vi "Process_day_file_strat.vi"(2 "Filename":path=path "/G3_3 HD/EnFlo Data/Oct_2000/3_Oct") -> (6 "Day KW Hrs":dbl, 7 "Night KWHrs":dbl format="%.2f", 10 "Time":dbl)   [LabVIEW 2010]
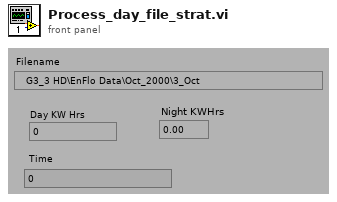
[diagram p1: front panel]
types:
  T1 = cluster{"second":i32, "minute":i32, "hour":i32, "day of month":i32, "month":i32, "year":i32, "day of week":i32, "day of year":i32, "is DST":i32}
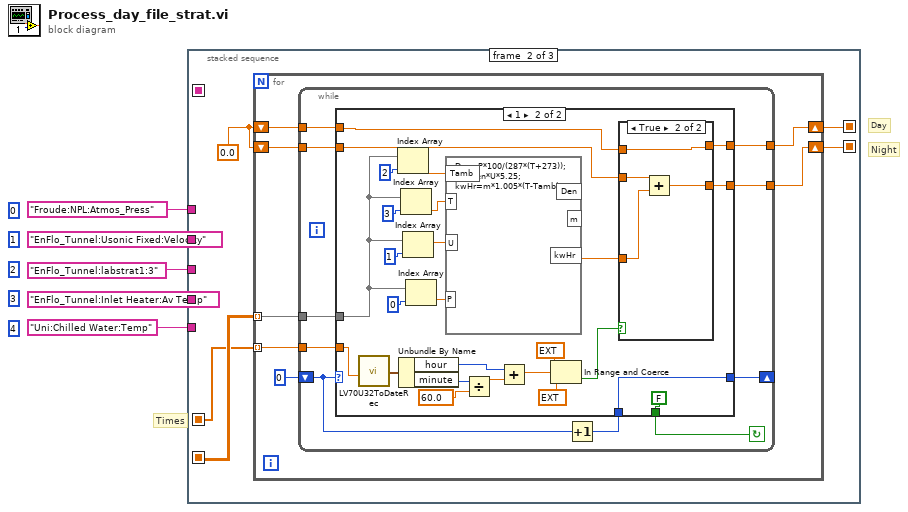
[diagram p0: block diagram]
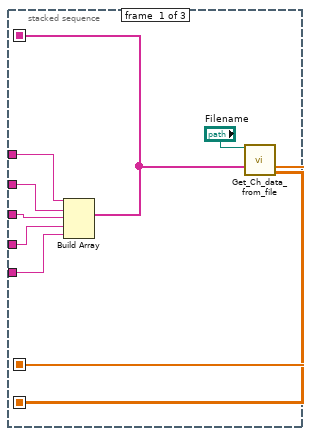
[diagram p2: hidden frame]
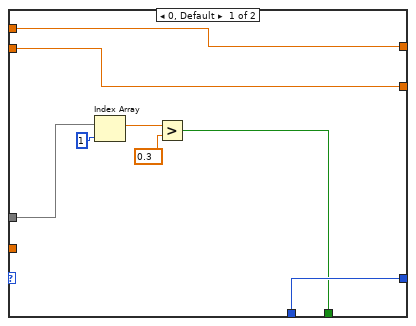
[diagram p3: hidden frame]
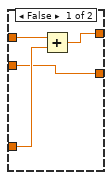
[diagram p4: hidden frame]
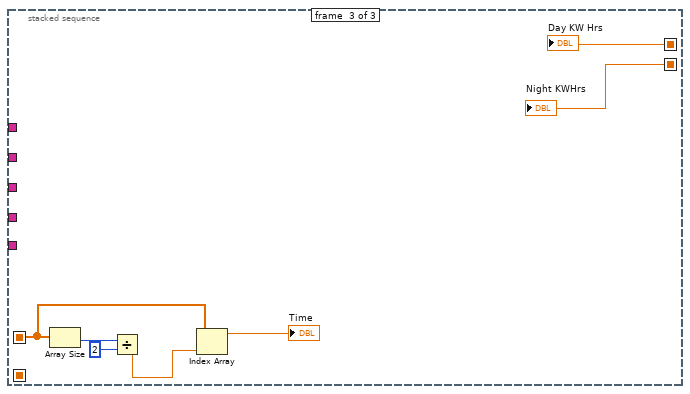
[diagram p5: hidden frame]
diagram:
  (unwired) 4
  (unwired) 3
  (unwired) 2
  (unwired) 1
  (unwired) 0
  # "Night"
  # "Day"
  # "Times"
  n1 = stacked-sequence {
    seq-local: [w8 _ _] -> [_ _ _]
    seq-local: [w7 _ _] -> [_ w17 w81]
    seq-local: [w6 _ _] -> [_ w19 _]
    seq-local: [_ w18 _] -> [_ _ w85]
    seq-local: [_ w15 _] -> [_ _ w79]
    tunnel: "Froude:NPL:Atmos_Press" -> [w14 _ _]
    tunnel: "EnFlo_Tunnel:Usonic Fixed:Velocity" -> [w13 _ _]
    tunnel: "EnFlo_Tunnel:labstrat1:3" -> [w12 _ _]
    tunnel: "EnFlo_Tunnel:Inlet Heater:Av Temp" -> [w11 _ _]
    tunnel: "Uni:Chilled Water:Temp" -> [w10 _ _]
    frame #0 {
      n2 = Build Array(w14, w13, w12, w11, w10) -> (w8:string[])
      n3 = call "Get_Ch_data_from_file.vi"("Filename"="Filename", "Channel names"=w8) -> ("Times"=w7:dbl[], "Ch Data"=w6:dbl[][])  [unwired: 10 in, 2 out]
    }
    frame #1 {
      w16 = 0.0
      n4 = for {
        tunnel: w19 -> [w25] mode=indexing
        shift-right: [w24] -> w18
        shift-left: w16 -> [w23]
        shift-right: [w20] -> w15
        shift-left: w16 -> [w21]
        tunnel: w17 -> [w22] mode=indexing
        n5 = while {
          tunnel: [w27] -> w20
          tunnel: w21 -> [w28]
          tunnel: w22 -> [w29]
          tunnel: w23 -> [w30]
          tunnel: [w31] -> w24
          tunnel: w25 -> [w36]
          shift-left: 0 -> [w34]
          shift-right: [w32] -> _
          stop <- w35 continue-if-true
          n6 = Increment(x=w34) -> (x+1=w33:i32)
          n7 = case shown="1" w34 {
            tunnel: w36 -> [w38 w66]
            tunnel: [w37 FALSE] -> w35
            tunnel: w33 -> [w41 w57]
            tunnel: [w41 w57] -> w32
            tunnel: [w40 w59] -> w31
            tunnel: w30 -> [w40 w60]
            tunnel: w29 -> [_ w56]
            tunnel: w28 -> [w39 w51]
            tunnel: [w39 w50] -> w27
            frame 0, Default {
              n8 = Index Array(array=w38, index=1 ("Index")) -> (element=w43:dbl)
              n9 = Greater?(x=w43, y=0.3) -> (0:w37:bool)
            }
            frame 1 {
              n10 = call <vilib>:"LV70U32ToDateRec.vi"("Time"=w56) -> ("date time rec"=w55:T1)
              n11 = Index Array(array=w66, index=2 ("Index")) -> (element=w62:dbl)
              n12 = Unbundle By Name(w55) -> ("hour"=w46:i32, "minute"=w49:i32)
              n13 = Index Array(array=w66, index=3 ("Index")) -> (element=w63:dbl)
              n14 = Index Array(array=w66, index=1 ("Index")) -> (element=w64:dbl)
              n15 = Index Array(array=w66, index=0 ("Index")) -> (element=w65:dbl)
              n16 = formula code="Den=P*100/(287*(T+273));\nm=Den*U*5.25;\nkwHr=m*1.005*(T-Tamb)/30;"("Tamb"=w62, "T"=w63, "U"=w64, "P"=w65) -> ("kwHr"=w61:dbl)  [unwired: 2 out]
              n17 = Divide(x=w49, y=60.0) -> (x/y=w47:dbl)
              n18 = Add(x=w46, y=w47) -> (x+y=w45:dbl)
              n19 = In Range and Coerce(upper limit=ext 7.5 ("hi"), x=w45, lower limit=ext 0.5 ("lo")) -> (In Range?=w52:bool)  [unwired: 1 out]
              n20 = case shown="True" w52 {
                tunnel: w61 -> [w74 w76]
                tunnel: w60 -> [w73 w78]
                tunnel: [w72 w78] -> w59
                tunnel: w51 -> [w71 w77]
                tunnel: [w71 w75] -> w50
                frame False {
                  n21 = Add(x=w73, y=w74) -> (x+y=w72:dbl)
                }
                frame True {
                  n22 = Add(x=w77, y=w76) -> (x+y=w75:dbl)
                }
              }
            }
          }
        }
      }
    }
    frame #2 {
      n23 = Array Size(array=w81) -> (size(s)=w84:i32)
      n24 = Divide(x=w84, y=2) -> (x/y=w82:dbl)
      n25 = Index Array(array=w81, index=w82) -> (element=→"Time":dbl)
      "Day KW Hrs" <- w85
      "Night KWHrs" <- w79
    }
  }
